vi "Running Average GUID Lookup.vi"() -> ()   [LabVIEW 2012, in "Running Average Custom Device.lvlib"]
doc: "Use this Global VI to access the GUIDs assigned to the page resources of the Custom Device."
uses:
  Running Average Custom Device.lvlib
panel:
  in  "Custom Device":string="164b0a39-1095-41b5-a00e-e1a471e58f47"
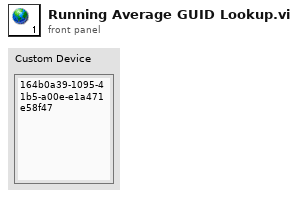
[diagram p1: front panel]
diagram:
